vi "GetValueFromCtrl.vi"(2 "imagesize":u32, 3 "new pixelsize ctrl":refnum<vi>) -> (0 "value":i32, 1 "new image dim":i32)   [LabVIEW 2009]
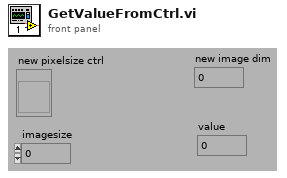
[diagram p1: front panel]
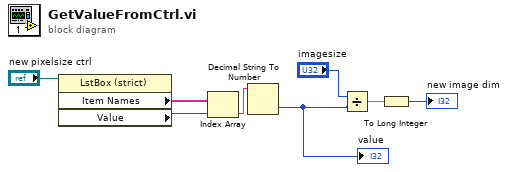
[diagram p0: block diagram]
diagram:
  n1 = property on="Property Node" class="LstBox (strict)"(reference="new pixelsize ctrl") -> ("Item Names"=w6:string[], "Value"=w7:i32)  [unwired: 1 in, 2 out]
  n2 = Index Array(array=w6, index=w7) -> (element=w5:string)
  n3 = Decimal String To Number(string=w5) -> (number=w4:i32)  [unwired: 2 in, 1 out]
  "value" <- w4
  n4 = Divide(x="imagesize", y=w4) -> (x/y=w3:dbl)
  n5 = To Long Integer(number=w3) -> (32bit integer=→"new image dim":i32)
